vi "DT3120_PassthruModes.vi"(11 "Modes":u32) -> (0 "DoesAsyncPassthruDirect":bool, 1 "DoesAsyncPassthru":bool, 2 "DoesSyncPassthruDirect":bool, 3 "DoesSyncPassthru":bool)   [LabVIEW 2010]
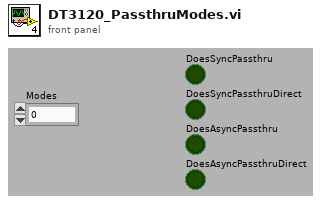
[diagram p1: front panel]
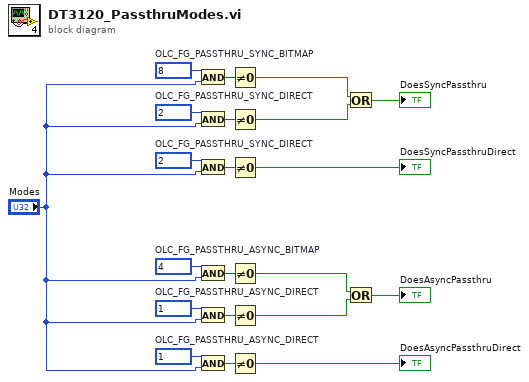
[diagram p0: block diagram]
diagram:
  w11 = u32 1  # OLC_FG_PASSTHRU_ASYNC_DIRECT
  w13 = u32 1  # OLC_FG_PASSTHRU_ASYNC_DIRECT
  w15 = u32 4  # OLC_FG_PASSTHRU_ASYNC_BITMAP
  w17 = u32 2  # OLC_FG_PASSTHRU_SYNC_DIRECT
  w19 = u32 2  # OLC_FG_PASSTHRU_SYNC_DIRECT
  w21 = u32 8  # OLC_FG_PASSTHRU_SYNC_BITMAP
  n1 = And(x=w21, y="Modes") -> (x .and. y?=w20:u32)
  n2 = And(x=w19, y="Modes") -> (x .and. y?=w18:u32)
  n3 = And(x=w17, y="Modes") -> (x .and. y?=w16:u32)
  n4 = And(x=w15, y="Modes") -> (x .and. y?=w14:u32)
  n5 = And(x=w13, y="Modes") -> (x .and. y?=w12:u32)
  n6 = And(x=w11, y="Modes") -> (x .and. y?=w10:u32)
  n7 = Not Equal To 0?(x=w20) -> (x != 0?=w8:bool)
  n8 = Not Equal To 0?(x=w18) -> (x != 0?=w7:bool)
  n9 = Not Equal To 0?(x=w16) -> (x != 0?=→"DoesSyncPassthruDirect":bool)
  n10 = Not Equal To 0?(x=w14) -> (x != 0?=w6:bool)
  n11 = Not Equal To 0?(x=w12) -> (x != 0?=w5:bool)
  n12 = Not Equal To 0?(x=w10) -> (x != 0?=→"DoesAsyncPassthruDirect":bool)
  n13 = Or(x=w8, y=w7) -> (x .or. y?=→"DoesSyncPassthru":bool)
  n14 = Or(x=w6, y=w5) -> (x .or. y?=→"DoesAsyncPassthru":bool)
